vi "Pre Launch Init.vi"(11 "Person in":refnum<class "Person.lvclass">) -> (0 "error out":errorcluster, 3 "Person out":refnum<class "Person.lvclass">)   [LabVIEW 2023, in "Person.lvlib" / "Person.lvclass"]
doc: "(<B>Filename</B>: Actor Framework.lvlib:Actor.lvclass:Pre Launch Init.vi)\n\nDefines behavior that occurs after the Launch Nested Actor method is invoked but before the actor's Actor Core method begins running.\n\nBy default, this method does nothing. A descendant class may override it to define behavior."
uses:
  Person.lvclass
  Person.lvclass/Person.ctl
  <vilib>/ActorFramework/Actor/Actor.lvclass
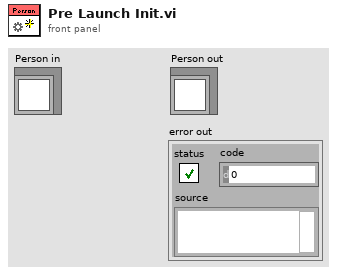
[diagram p1: front panel]
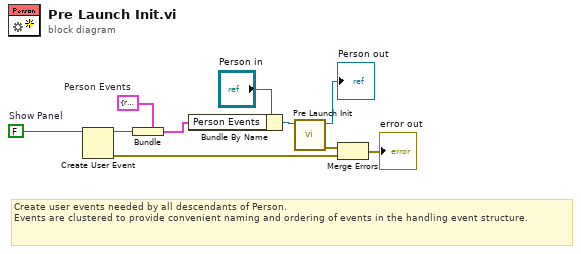
[diagram p0: block diagram]
diagram:
  w1 = cluster{"Show Panel":refnum<user-event>} {"Show Panel"=refnum}  # Person Events
  w9 = FALSE  # Show Panel
  # "Create user events needed by all descendants of Person.\nEvents are clustered to provide convenient naming and ordering of events in the handling event structure."
  n1 = Create User Event(user event datatype=w9) -> (user event=w3:refnum<user-event>, error out=w4:errorcluster)  [unwired: 1 in]
  n2 = Bundle(cluster=w1, "Show Panel"=w3) -> (w2:cluster{"Show Panel":refnum<user-event>})
  n3 = Bundle By Name(cluster="Person in", "Person Events"=w2) -> (w7:refnum<class "Person.lvclass">)
  n4 = call-parent "Pre Launch Init.vi"("Actor in"=w7) -> ("error out"=w6:errorcluster, "Actor out"=→"Person out":refnum<class "Person.lvclass">)  [unwired: 9 in]
  n5 = Merge Errors(w6, w4) -> (→"error out":errorcluster)
